vi "isDone.vi"(8 "error in (no error)":errorcluster, 11 "TrapezoidalWave in":refnum<class "TrapezoidalWave.lvclass">) -> (0 "error out":errorcluster, 2 "isDone?":bool=TRUE, 3 "TrapezoidalWave out":refnum<class "TrapezoidalWave.lvclass">)   [LabVIEW 2015, in "TrapezoidalWave.lvclass"]
uses:
  TrapezoidalWave.lvclass
  TrapezoidalWave.lvclass/TrapezoidalWave.ctl
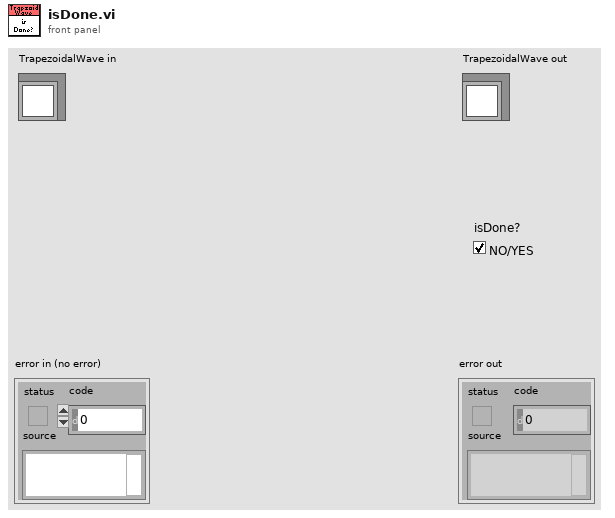
[diagram p1: front panel]
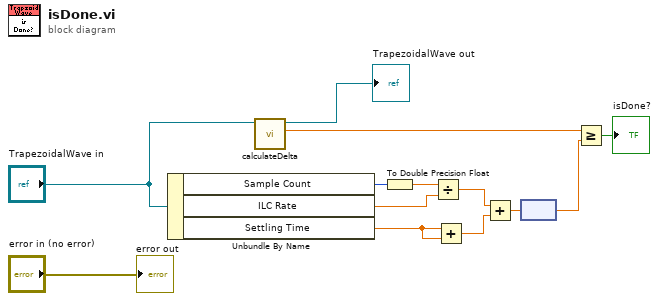
[diagram p0: block diagram]
diagram:
  n1 = Unbundle By Name("TrapezoidalWave in") -> ("Sample Count"=w8:u32, "ILC Rate"=w6:dbl[unit], "Settling Time"=w5:dbl[unit])
  n2 = call "calculateDelta.vi"("TrapezoidalWave in"="TrapezoidalWave in") -> ("Delta Timestamp"=w11:dbl, "TrapezoidalWave out"=→"TrapezoidalWave out":refnum<class "TrapezoidalWave.lvclass">)  [unwired: 8 in, 1 out]
  n3 = To Double Precision Float(number=w8) -> (double precision float=w7:dbl)
  n4 = Divide(x=w7, y=w6) -> (x/y=w4:dbl[unit])
  n5 = Add(x=w5, y=w5) -> (x+y=w3:dbl[unit])
  n6 = Add(x=w4, y=w3) -> (x+y=w2:dbl[unit])
  n7 = node(w2) -> (w1:dbl)
  n8 = Greater Or Equal?(x=w11, y=w1) -> (x >= y?=→"isDone?":bool)
  "error out" <- "error in (no error)"
